vi "_Run Cycle.vi"(3 "Init (F)":bool, 4 "Update":bool) -> (0 "LC Input Detected":bool, 1 "Finish Run?":bool)   [LabVIEW 2015]
uses:
  <vilib>/rvi/Emulation/niFpgaGetClockAttributes.vi
  <vilib>/rvi/Emulation/niFpgaSctlEmulationGetInTimedLoop.vi
  <vilib>/rvi/Emulation/niFpgaEmulationReportErrorSimple.vi
  Instance           9 18Saved   _Run Cycle .vi
  <vilib>/rvi/Memory/Memory_Emulation/nirvimemoryEmulation.vi
  <vilib>/rvi/Memory/Memory_Emulation/nirvimemoryFastEmulation.vi
  <vilib>/rvi/DataTransferAndStorage/Container/Common/niFpgaContainerGetUniqueNameForEmu.vi
  <vilib>/rvi/Memory/Memory_Emulation/niFpgaMemoryEmulationCacheClearOnFirstRun.vi
  <vilib>/rvi/Memory/Memory_Emulation/nirvimemoryEmulationManagerCache_MakeExclusive.vi
  <vilib>/rvi/Memory/Memory_Emulation/niFpgaMemoryEmulationValidateCache.vi
  <vilib>/rvi/Memory/Memory_Emulation/nirvimemoryEmulationManagerCache_InsertValue.vi
  <vilib>/Utility/error.llb/Clear Errors.vi
  <vilib>/rvi/Memory/Memory_Emulation/nirvimemoryEmulationManagerCache_ReleaseExclusive.vi
  <vilib>/rvi/Memory/Memory_Emulation/nirvimemoryEmulationManagerCache_GetValue.vi
  <vilib>/rvi/Emulation/niFpgaEmulationIsFPGAContextNoSignature.vi
  <vilib>/rvi/Memory/Memory_Emulation/nirvimemoryEmulationManagerCache_SetValue.vi
  <vilib>/rvi/Emulation/niFpgaSctlEmulationResourceMgr.vi
  <vilib>/rvi/Emulation/niFpgaCriticalErrorInLSC.vi
  <vilib>/rvi/Emulation/niFpgaProcessEmulError.vi
  <vilib>/rvi/DataTransferAndStorage/Container/XNode/niFpgaContainer.xnode
  <vilib>/rvi/DataTransferAndStorage/Register/Emulation/niFpgaRegisterEmulation.vi
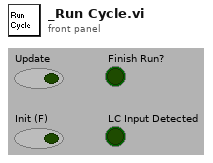
[diagram p1: front panel]
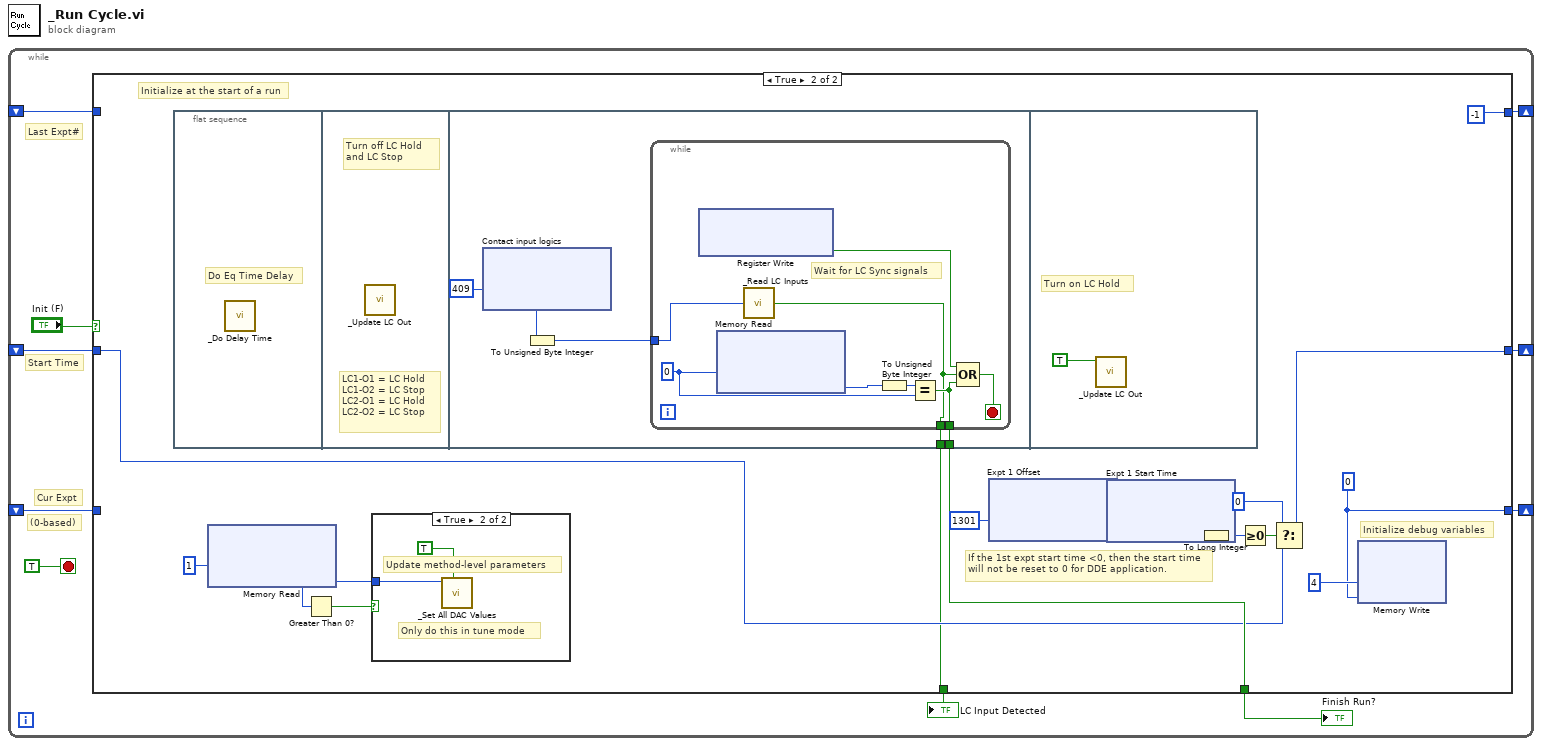
[diagram p0: block diagram]
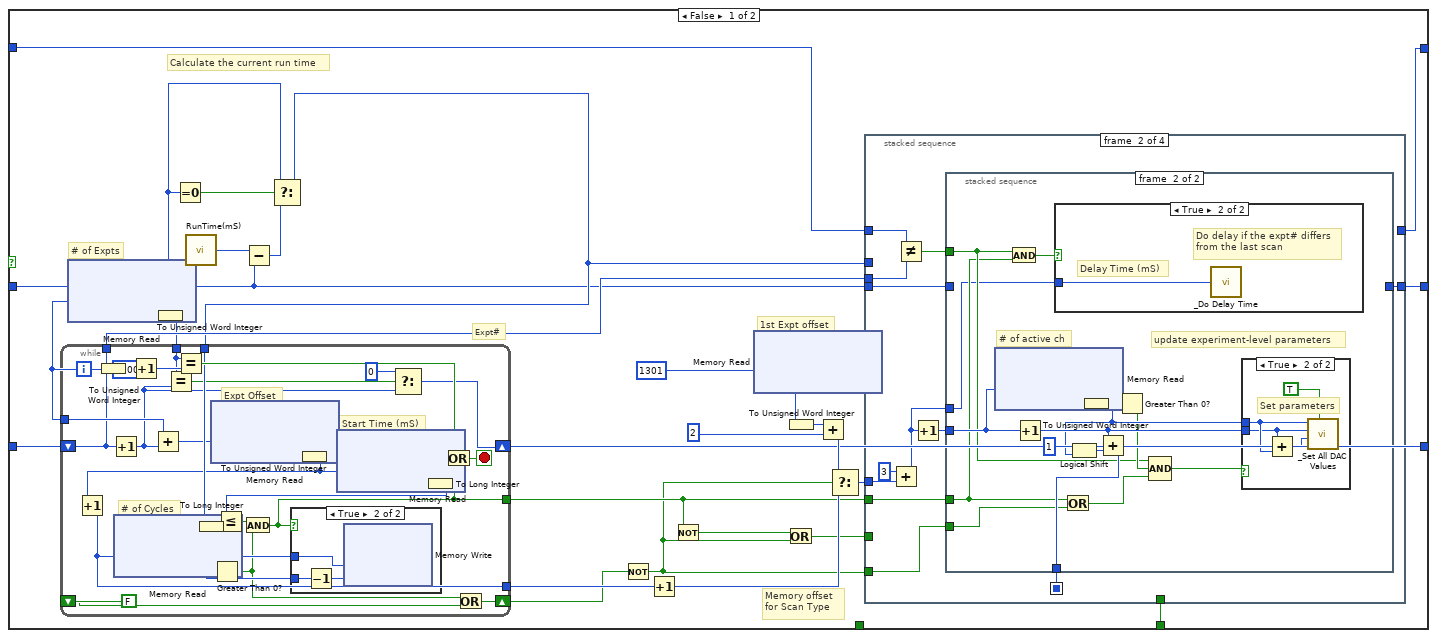
[diagram p2: hidden frame]
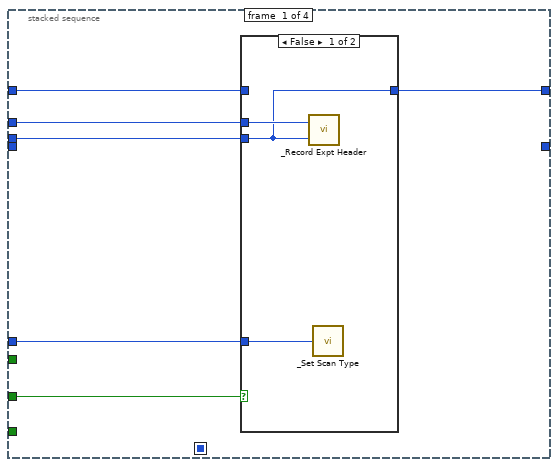
[diagram p3: hidden frame]
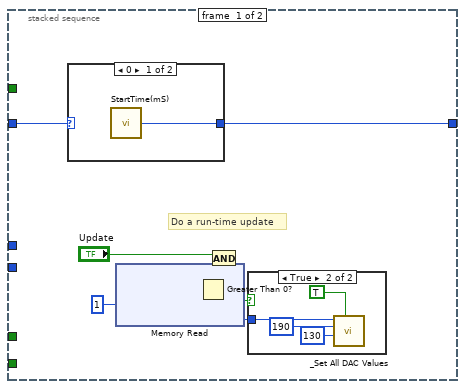
[diagram p5: hidden frame]
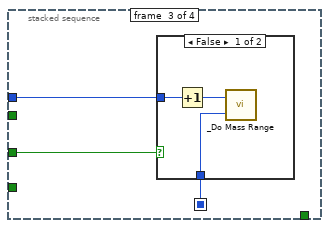
[diagram p10: hidden frame]
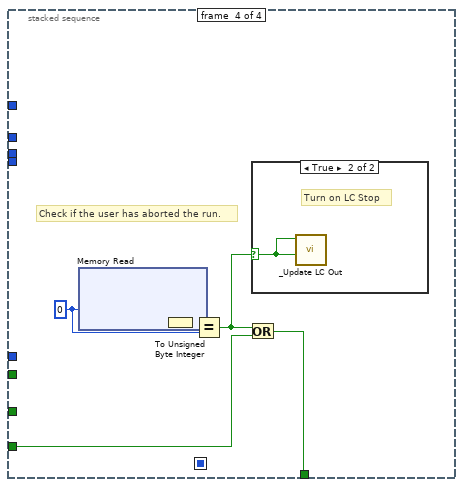
[diagram p12: hidden frame]
diagram:
  n1 = while {
    shift-right: [w9] -> _
    shift-left: _ -> [w8]
    shift-right: [w6] -> _
    shift-left: _ -> [w5]
    shift-right: [w3] -> _
    shift-left: _ -> [w2]
    stop <- TRUE stop-if-true
    # "Last Expt#"
    # "(0-based)"
    # "Cur Expt"
    # "Start Time"
    n2 = case shown="True" "Init (F)" {
      tunnel: [w14 w139] -> w9
      tunnel: w8 -> [w15 w140]
      tunnel: [w26 w142] -> w6
      tunnel: w5 -> [w29 _]
      tunnel: [w27 w150] -> w4
      tunnel: [w11 i16 -1 ("Data")] -> w3
      tunnel: w2 -> [w12 _]
      tunnel: [_ w137] -> w1
      frame False {
        w38 = u16 1300 ("Address")
        # "Calculate the current run time"
        # "Memory offset\nfor Scan Type"
        # "1st Expt offset"
        # "# of Expts"
        # "Expt#"
        n3 = xnode ("Memory Read")("Address"=w38) -> ("Data"=w37:u32)  [unwired: 1 in, 1 out]
        n4 = To Unsigned Word Integer(number=w37) -> (unsigned 16bit integer=w13:u16)
        n5 = Equal To 0?(x=w15) -> (x = 0?=w18:bool)
        n6 = call "RunTime(mS)"() -> ("Tick Count(mSec)"=w28:u32)
        n7 = Subtract(x=w28, y=w15) -> (x-y=w17:u32)
        n8 = Select(t=w15, s=w18, f=w17) -> (s? t:f=w16:u32)
        n9 = while {
          tunnel: w16 -> [w130]
          shift-right: [w120] -> w26
          shift-left: w29 -> [w115]
          tunnel: [w117] -> w39
          tunnel: w13 -> [w123]
          tunnel: w38 -> [w126]
          tunnel: [w115] -> w25
          shift-right: [w114] -> w23
          shift-left: FALSE -> [w113]
          tunnel: [w111] -> w21
          i -> [w129]
          stop <- w132 stop-if-true
          # "# of Cycles"
          # "Start Time (mS)"
          # "Expt Offset"
          n10 = To Unsigned Word Integer(number=w129) -> (unsigned 16bit integer=w125:u16)
          n11 = Increment(x=w115) -> (x+1=w116:u16)
          n12 = Increment(x=w125) -> (x+1=w124:u16)
          n13 = Add(x=w126, y=w116) -> (x+y=w128:u16)
          n14 = Equal?(x=w123, y=w116) -> (x = y?=w122:bool)
          n15 = Equal?(x=w123, y=w124) -> (x = y?=w131:bool)
          n16 = To Long Integer(number=w130) -> (32bit integer=w108:i32)
          n17 = xnode ("Memory Read")("Address"=w128) -> ("Data"=w127:u32)  [unwired: 1 in, 1 out]
          n18 = To Unsigned Word Integer(number=w127) -> (unsigned 16bit integer=w119:u16)
          n19 = Increment(x=w119) -> (x+1=w117:u16)
          n20 = xnode ("Memory Read")("Address"=w117) -> ("Data"=w118:u32)  [unwired: 1 in, 1 out]
          n21 = Greater Than 0?(x=w118) -> (x > 0?=w112:bool)
          n22 = xnode ("Memory Read")("Address"=w119) -> ("Data"=w110:u32)  [unwired: 1 in, 1 out]
          n23 = Select(t=u16 0, s=w122, f=w116) -> (s? t:f=w120:u16)
          n24 = To Long Integer(number=w110) -> (32bit integer=w109:i32)
          n25 = Less Or Equal?(x=w109, y=w108) -> (x <= y?=w133:bool)
          n26 = And(x=w133, y=w112) -> (x .and. y?=w111:bool)
          n27 = case shown="True" w111 {
            tunnel: w118 -> [_ w135]
            tunnel: w117 -> [_ w136]
            frame False {
            }
            frame True {
              n28 = Decrement(x=w135) -> (x-1=w134:u32)
              n29 = xnode ("Memory Write")("Address"=w136, "Data"=w134) -> ()  [unwired: 1 in, 1 out]
            }
          }
          n30 = Or(x=w131, y=w111) -> (x .or. y?=w132:bool)
          n31 = Or(x=w112, y=w113) -> (x .or. y?=w114:bool)
        }
        n32 = Not(x=w23) -> (.not. x?=w20:bool)
        n33 = Increment(x=w39) -> (x+1=w30:u16)
        n34 = Not(x=w21) -> (.not. x?=w22:bool)
        n35 = xnode ("Memory Read")("Address"=u16 1301) -> ("Data"=w34:u32)  [unwired: 1 in, 1 out]
        n36 = To Unsigned Word Integer(number=w34) -> (unsigned 16bit integer=w33:u16)
        n37 = Or(x=w22, y=w20) -> (x .or. y?=w19:bool)
        n38 = Add(x=w33, y=u8 2) -> (x+y=w32:u16)
        n39 = Select(t=w32, s=w20, f=w30) -> (s? t:f=w31:u16)
        n40 = stacked-sequence {
          seq-local: [_ w60 _ _] -> [_ _ w97 _]
          tunnel: w16 -> [w42 _ _ _]
          tunnel: w25 -> [w45 w51 _ _]
          tunnel: w31 -> [w43 w55 w96 _]
          tunnel: w20 -> [_ w56 _ w103]
          tunnel: [_ _ _ w102] -> w27
          tunnel: w21 -> [_ w57 _ _]
          tunnel: w19 -> [w44 _ w95 _]
          tunnel: w15 -> [_ w54 _ _]
          tunnel: [_ w53 _ _] -> w14
          tunnel: w12 -> [w41 w52 _ _]
          tunnel: [w40 _ _ _] -> w11
          frame #0 {
            n41 = case shown="False" w44 {
              tunnel: w42 -> [w47 _]
              tunnel: w45 -> [w46 _]
              tunnel: w43 -> [w48 _]
              tunnel: w41 -> [_ w49]
              tunnel: [w46 w49] -> w40
              frame False {
                n42 = call "_Record Expt Header.vi"("Expt/Cycle#"=w46, "Run Time (mS)"=w47) -> ()  [unwired: 1 out]
                n43 = call "_Set Scan Type.vi"("ScanType Offset"=w48) -> ()
              }
              frame True {
                # "Pause period or finish run."
              }
            }
          }
          frame #1 {
            n44 = Add(x=u8 3, y=w55) -> (x+y=w58:u16)
            n45 = Not Equal?(x=w52, y=w51) -> (x != y?=w50:bool)
            n46 = Increment(x=w58) -> (x+1=w61:u16)
            n47 = stacked-sequence {
              tunnel: w61 -> [_ w89]
              tunnel: [_ w88] -> w60
              tunnel: w58 -> [_ w75]
              tunnel: w57 -> [_ w77]
              tunnel: w56 -> [_ w87]
              tunnel: w54 -> [w68 _]
              tunnel: [w67 _] -> w53
              tunnel: w50 -> [_ w78]
              frame #0 {
                # "Do a run-time update"
                n48 = case shown="0" w68 {
                  selector: w68 -> [_ w74]
                  tunnel: [w73 w74] -> w67
                  frame 0 {
                    n49 = call "StartTime(mS)"() -> ("Tick Count(mSec)"=w73:u32)
                  }
                  frame 1, Default {
                  }
                }
                n50 = xnode ("Memory Read")("Address"=u8 1) -> ("Data"=w63:u32)  [unwired: 1 in, 1 out]
                n51 = Greater Than 0?(x=w63) -> (x > 0?=w65:bool)
                n52 = And(x="Update", y=w65) -> (x .and. y?=w64:bool)
                n53 = case shown="True" w64 {
                  tunnel: w63 -> [_ w70]
                  frame False {
                  }
                  frame True {
                    n54 = call "_Set All DAC Values.vi"("Record Values (F)"=TRUE, "DAC Value Offset (70)"=u16 130 ("DAC Value Offset (110)"), "Channel ID Offset (10)"=u16 190, "# of Active Channels"=w70) -> ()  [unwired: 5 in]
                  }
                }
              }
              frame #1 {
                # "update experiment-level parameters"
                # "# of active ch"
                n55 = xnode ("Memory Read")("Address"=w89) -> ("Data"=w83:u32)  [unwired: 1 in, 1 out]
                n56 = And(x=w78, y=w77) -> (x .and. y?=w76:bool)
                n57 = Increment(x=w89) -> (x+1=w84:u16)
                n58 = case shown="True" w76 {
                  tunnel: w75 -> [_ w90]
                  frame False {
                    # "No Pause for Subsequent Cycles\nor single experiment method"
                  }
                  frame True {
                    # "Delay Time (mS)"
                    # "Do delay if the expt# differs\nfrom the last scan"
                    n59 = call "_Do Delay Time.vi"("DelayTime Address"=w90) -> ()
                  }
                }
                n60 = Or(x=w77, y=w87) -> (x .or. y?=w79:bool)
                n61 = To Unsigned Word Integer(number=w83) -> (unsigned 16bit integer=w82:u16)
                n62 = Logical Shift(y=u8 1, x=w82) -> (x << y=w85:u16)
                n63 = Add(x=w84, y=w85) -> (x+y=w88:u16)
                n64 = Greater Than 0?(x=w82) -> (x > 0?=w81:bool)
                n65 = Compound Arithmetic op=AND(w78, w81, w79) -> (w80:bool)
                n66 = case shown="True" w80 {
                  tunnel: w82 -> [_ w93]
                  tunnel: w84 -> [_ w92]
                  frame False {
                    # "Pause Period"
                  }
                  frame True {
                    # "Set parameters"
                    n67 = Add(x=w92, y=w93) -> (x+y=w94:u16)
                    n68 = call "_Set All DAC Values.vi"("Record Values (F)"=TRUE, "DAC Value Offset (70)"=w94, "Channel ID Offset (10)"=w92, "# of Active Channels"=w93) -> ()  [unwired: 5 in]
                  }
                }
              }
            }
          }
          frame #2 {
            n69 = case shown="False" w95 {
              tunnel: w97 -> [w100 _]
              tunnel: w96 -> [w99 _]
              frame False {
                n70 = Increment(x=w99) -> (x+1=w98:u16)
                n71 = call "_Do Mass Range.vi"("# of MR Offset"=w100, "Pause Time Offset"=w98) -> ()  [unwired: 2 out]
              }
              frame True {
                # "Pause Period\nor Finish Run"
              }
            }
          }
          frame #3 {
            w106 = u8 0 ("Address")
            # "Check if the user has aborted the run."
            n72 = xnode ("Memory Read")("Address"=w106) -> ("Data"=w104:u32)  [unwired: 1 in, 1 out]
            n73 = To Unsigned Byte Integer(number=w104) -> (unsigned 8bit integer=w105:u8)
            n74 = Equal?(x=w105, y=w106) -> (x = y?=w101:bool)
            n75 = Or(x=w101, y=w103) -> (x .or. y?=w102:bool)
            n76 = case shown="True" w101 {
              selector: w101 -> [_ w107]
              frame False {
              }
              frame True {
                # "Turn on LC Stop"
                n77 = call "_Update LC Out.vi"("LC Stop"=w107, "LC Hold"=w107) -> ()  [unwired: 6 out]
              }
            }
          }
        }
      }
      frame True {
        w142 = u16 0 ("Data")
        # "If the 1st expt start time <0, then the start time\nwill not be reset to 0 for DDE application."
        # "Initialize debug variables"
        # "Initialize at the start of a run"
        n78 = flat-sequence {
          tunnel: [w159] -> w150
          tunnel: [w155] -> w137
          frame #0 {
            # "Do Eq Time Delay"
            n79 = call "_Do Delay Time.vi"() -> ()  [unwired: 1 in]
          }
          frame #1 {
            # "Turn off LC Hold \nand LC Stop"
            # "LC1-O1 = LC Hold\nLC1-O2 = LC Stop\nLC2-O1 = LC Hold\nLC2-O2 = LC Stop"
            n80 = call "_Update LC Out.vi"() -> ()  [unwired: 2 in, 6 out]
          }
          frame #2 {
            n81 = xnode "Contact input logics"("Address"=u16 409) -> ("Data"=w157:u32)  [unwired: 1 in, 1 out]
            n82 = To Unsigned Byte Integer(number=w157) -> (unsigned 8bit integer=w156:u8)
            n83 = while {
              tunnel: [w164] -> w159
              tunnel: w156 -> [w162]
              tunnel: [w160] -> w155
              stop <- w165 stop-if-true
              w166 = u8 0 ("Address")
              # "Wait for LC Sync signals"
              n84 = xnode "Register Write"() -> ("Data"=w161:bool)  [unwired: 1 in, 1 out]
              n85 = xnode ("Memory Read")("Address"=w166) -> ("Data"=w167:u32)  [unwired: 1 in, 1 out]
              n86 = call "_Read LC Inputs.vi"("LogicOption"=w162) -> ("LC Input Detected"=w160:bool)
              n87 = To Unsigned Byte Integer(number=w167) -> (unsigned 8bit integer=w163:u8)
              n88 = Equal?(x=w163, y=w166) -> (x = y?=w164:bool)
              n89 = Compound Arithmetic op=OR(w161, w160, w164) -> (w165:bool)
            }
          }
          frame #3 {
            # "Turn on LC Hold"
            n90 = call "_Update LC Out.vi"("LC Hold"=TRUE ("Port5/DIO5")) -> ()  [unwired: 1 in, 6 out]
          }
        }
        n91 = xnode ("Memory Read")("Address"=u8 1) -> ("Data"=w149:u32)  [unwired: 1 in, 1 out]
        n92 = Greater Than 0?(x=w149) -> (x > 0?=w148:bool)
        n93 = case shown="True" w148 {
          tunnel: w149 -> [_ w154]
          frame False {
          }
          frame True {
            # "Update method-level parameters"
            # "Only do this in tune mode"
            n94 = call "_Set All DAC Values.vi"("Record Values (F)"=TRUE, "# of Active Channels"=w154) -> ()  [unwired: 7 in]
          }
        }
        n95 = xnode "Expt 1 Offset"("Address"=u16 1301) -> ("Data"=w146:u32)  [unwired: 1 in, 1 out]
        n96 = xnode "Expt 1 Start Time"("Address"=w146) -> ("Data"=w145:u32)  [unwired: 1 in, 1 out]
        n97 = To Long Integer(number=w145) -> (32bit integer=w144:i32)
        n98 = Greater Or Equal To 0?(x=w144) -> (x >= 0?=w143:bool)
        n99 = Select(t=u32 0 ("Tick Count(mSec)"), s=w143, f=w140) -> (s? t:f=w139:u32)
        n100 = xnode ("Memory Write")("Address"=u8 4, "Data"=w142) -> ()  [unwired: 1 in, 1 out]
      }
    }
    "Finish Run?" <- w4
    "LC Input Detected" <- w1
  }
